vi "Disconnect.vi"(8 "error in (no error)":errorcluster, 11 "TCP slave instance":refnum<class "Modbus Slave.lvclass">) -> ()   [LabVIEW 2021]
uses:
  <vilib>/Modbus/slave/Modbus Slave.lvclass
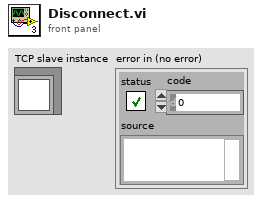
[diagram p1: front panel]
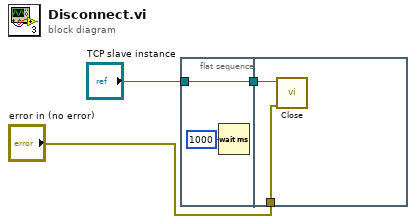
[diagram p0: block diagram]
diagram:
  n1 = flat-sequence {
    tunnel: "TCP slave instance" -> [w5]
    tunnel: [w5] -> w3
    tunnel: w3 -> [w7]
    tunnel: "error in (no error)" -> [w6]
    frame #0 {
      n2 = Wait (ms)(milliseconds to wait=u32 1000) -> ()  [unwired: 1 out]
    }
    frame #1 {
      n3 = call-dynamic "Close.vi"("error in (no error)"=w6, "Modbus slave in"=w7) -> ()  [unwired: 9 in, 1 out]
    }
  }
